vi "Ultrasonic Analytic Code.vi"(11 "AIDeviceRef 2":T1={"DevStatus"={"status"=FALSE, "code"=0, "source"=""}, "Analog Module"=enum."Analog Module 1", "Analog Channel"=enum."Invalid"}) -> (2 "AIDeviceRef":T1, 3 "Distance":dbl)   [LabVIEW 2013]
uses:
  <vilib>/Rock Robotics/WPI/AnalogChannel/WPI_AnalogChannelDevRef.ctl
  <vilib>/Rock Robotics/SystemInterfaces/Typedef/FPGA_TypedefAnalogModule.ctl
  <vilib>/Rock Robotics/SystemInterfaces/AI/FPGA_AIChannel.ctl
panel:
  in  "Scaling factor (V/in)":dbl=0.0098
  in  "Samples Per Second":dbl=1000.0
  in  "Average Bits":u8=6 max=15
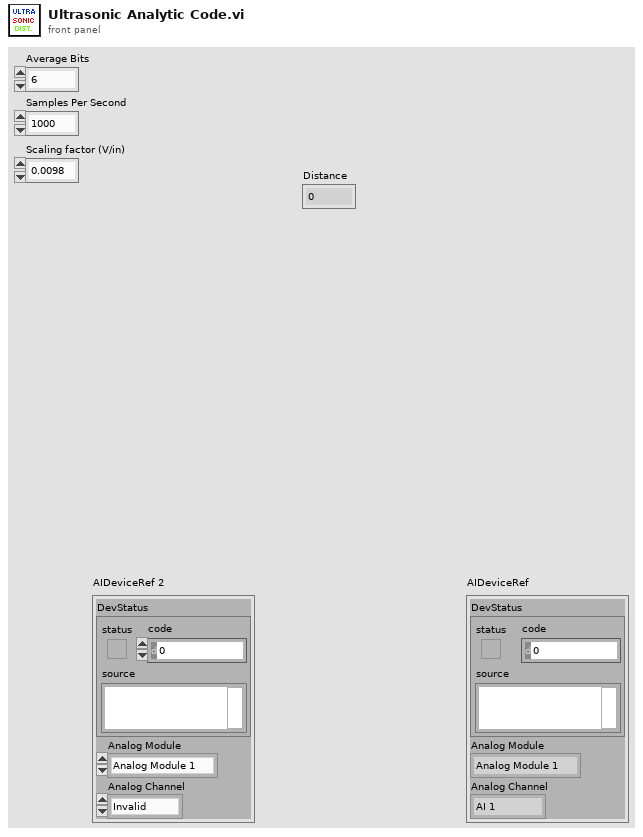
[diagram p1: front panel]
types:
  T1 = typedef "WPI_AnalogChannelDevRef.ctl" = cluster{"DevStatus":errorcluster, "Analog Module":T2, "Analog Channel":T3}
  T2 = typedef "FPGA_TypedefAnalogModule.ctl" = enum16{"Analog Module 1", "Analog Module 2"}
  T3 = typedef "FPGA_AIChannel.ctl" = enum8{"AI 1", "AI 2", "AI 3", "AI 4", "AI 5", "AI 6", "AI 7", "AI 8", "Invalid"}
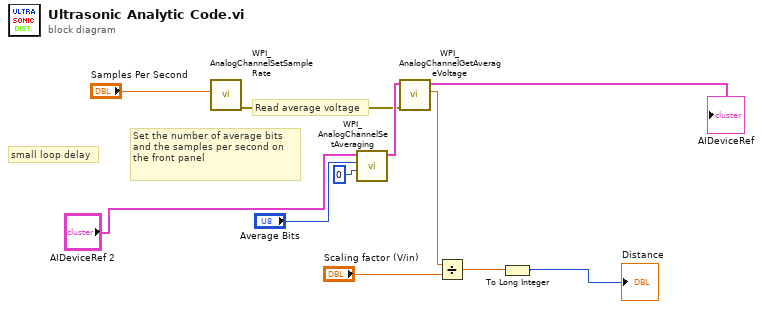
[diagram p0: block diagram]
diagram:
  # "small loop delay"
  # "Read average voltage"
  # "Set the number of average bits and the samples per second on the front panel"
  n1 = call <vilib>:"WPI_AnalogChannelSetSampleRate.vi"("Samples Per Second"="Samples Per Second") -> ("error out"=w5:errorcluster)  [unwired: 3 in, 7 out]
  n2 = call <vilib>:"WPI_AnalogChannelSetAveraging.vi"("OversampleBits"=u8 0, "AverageBits"="Average Bits", "AIDeviceRef"="AIDeviceRef 2") -> ("AIDeviceRef"=w6:T1)  [unwired: 1 in, 7 out]
  n3 = call <vilib>:"WPI_AnalogChannelGetAverageVoltage.vi"("error in (no error)"=w5, "AIDeviceRef"=w6) -> ("Voltage"=w7:dbl, "AIDeviceRef"=→"AIDeviceRef":T1)  [unwired: 8 out]
  n4 = Divide(x=w7, y="Scaling factor (V/in)") -> (x/y=w3:dbl)
  n5 = To Long Integer(number=w3) -> (32bit integer=→"Distance":i32)
